vi "element to byte index.vi"(7 "big endian?":bool, 9 "element number":i32, 10 "data type":T1, 11 "assembly size (bytes)":u32) -> (2 "subindex":i32, 3 "byte index":i32)   [LabVIEW 2013, in "EthernetIP Channel.lvclass"]
uses:
  EthernetIP Channel.lvclass
  <vilib>/NI/Tag Bus/tag/Data Type.ctl
  <vilib>/NI/Tag Bus/tag/tag descriptor.lvclass
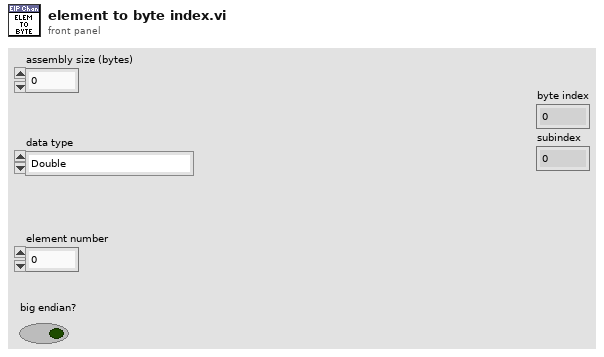
[diagram p1: front panel]
types:
  T1 = typedef "tag bus.lvlib/tag descriptor.lvclass/Data Type.ctl" = enum16{"Double", "Single", "I64", "I32", "I16", "I8", "U64", "U32", "U16", "U8", "Boolean", "String", "Array of Double", "Array of Single", "Array of I64", "Array of I32", "Array of I16", "Array of I8", "Array of U64", "Array of U32", "Array of U16", "Array of U8", "Array of Boolean", "Array of String"}
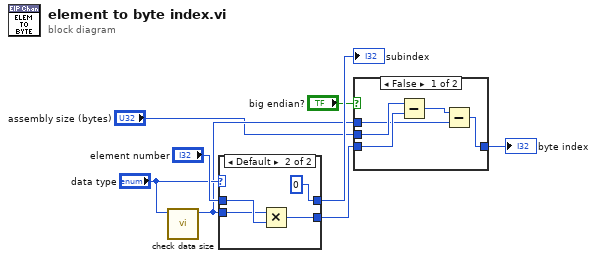
[diagram p0: block diagram]
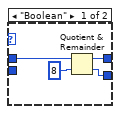
[diagram p3: hidden frame]
diagram:
  n1 = call "check data size.vi"("data type"="data type") -> ("bytes"=w2:i32)  [unwired: 10 in]
  n2 = case shown="Default" "data type" {
    tunnel: [w9 0 ("subindex 2")] -> w8
    tunnel: "element number" -> [w12 w15]
    tunnel: [w10 w14] -> w4
    tunnel: w2 -> [_ w13]
    frame "Boolean" {
      n3 = Quotient & Remainder(x=w12, y=8) -> (x-y*floor(x/y)=w9:i32, floor(x/y)=w10:i32)
    }
    frame Default {
      n4 = Multiply(x=w13, y=w15) -> (x*y=w14:i32)
    }
  }
  "subindex" <- w8
  n5 = case shown="False" "big endian?" {
    tunnel: [w17 w22] -> w5
    tunnel: w4 -> [w20 w22]
    tunnel: w2 -> [w19 _]
    tunnel: "assembly size (bytes)" -> [w21 _]
    frame False {
      n6 = Subtract(x=w21, y=w20) -> (x-y=w18:u32)
      n7 = Subtract(x=w18, y=w19) -> (x-y=w17:u32)
    }
    frame True {
    }
  }
  "byte index" <- w5
